vi "NI VeriStand - Get Custom Device Runtime Configuration Ref.vi"(8 "error in":errorcluster, 11 "Runtime Configuration Ref":refnum<k24>) -> (0 "error out":errorcluster, 2 "Parent Ref":T1 format="%.0x", 3 "Runtime Configuration Ref out":refnum<k24>)   [LabVIEW 2025]
uses:
  NationalInstruments.VeriStand.SystemDefinitionAPI
  <vilib>/NI VeriStand/Custom Device API/Custom Device Item Ref.ctl
  <vilib>/NI VeriStand/Custom Device API/Custom Device API.lvlib
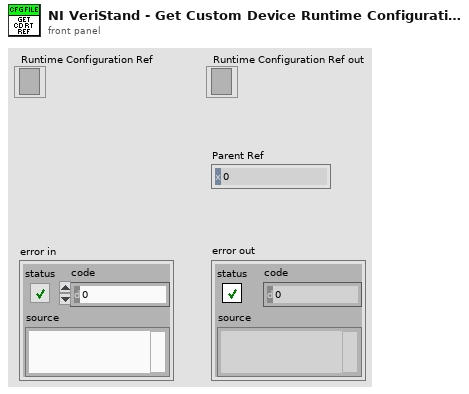
[diagram p1: front panel]
types:
  T1 = typedef "Custom Device API.lvlib/Custom Device Item Ref.ctl" = u64
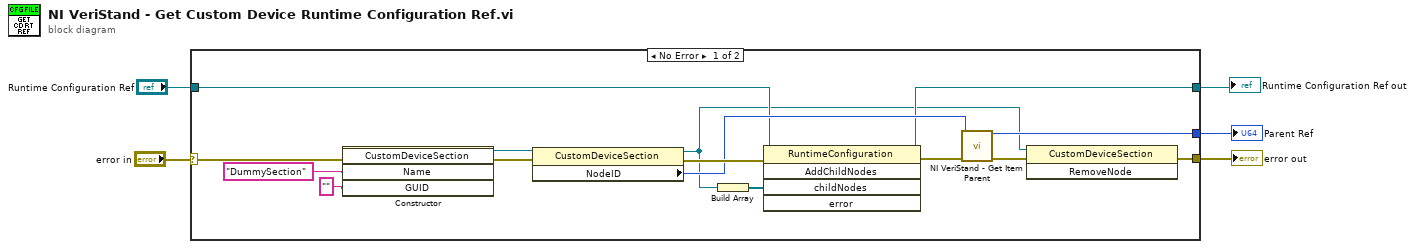
[diagram p0: block diagram]
diagram:
  n1 = case shown="No Error" "error in" {
    selector: "error in" -> [w17 w22]
    tunnel: "Runtime Configuration Ref" -> [w9 w21]
    tunnel: [w8 w21] -> w2
    tunnel: [w14 _] -> w1
    tunnel: [w19 w22] -> w5
    frame No Error {
      n2 = constructor class="CustomDeviceSection"(error in=w17, "Name"="DummySection", "GUID"="") -> (reference out=w10:refnum<k24>, error out=w18:errorcluster)  [unwired: 2 in, 3 out]
      n3 = property class="CustomDeviceSection"(reference=w10, error in=w18) -> (reference out=w7:refnum<k24>, error out=w16:errorcluster, "NodeID"=w13:u64)
      n4 = Build Array(w7) -> (w6:refnum<k24>[])
      n5 = invoke class="RuntimeConfiguration" method="AddChildNodes"(reference=w9, error in=w16, "childNodes"=w6) -> (reference out=w8:refnum<k24>, error out=w15:errorcluster)  [unwired: 2 in, 3 out]
      n6 = call <vilib>:"NI VeriStand - Get Item Parent.vi"("error in (no error)"=w15, "Item Ref in"=w13) -> ("error out"=w20:errorcluster, "Parent Ref"=w14:T1)  [unwired: 6 in, 2 out]
      n7 = invoke class="CustomDeviceSection" method="RemoveNode"(reference=w7, error in=w20) -> (error out=w19:errorcluster)  [unwired: 1 in, 2 out]
    }
    frame Error {
    }
  }
  "Parent Ref" <- w1
  "error out" <- w5
  "Runtime Configuration Ref out" <- w2
